vi "save file data.vi"(8 "error in":errorcluster, 10 "format":T1, 11 "Path":path) -> (0 "error out":errorcluster)   [LabVIEW 2013, in "NISE_CEF_TreeSerializer.lvlib"]
uses:
  NISE_CEF_TreeSerializer.lvlib
  base file format.ctl
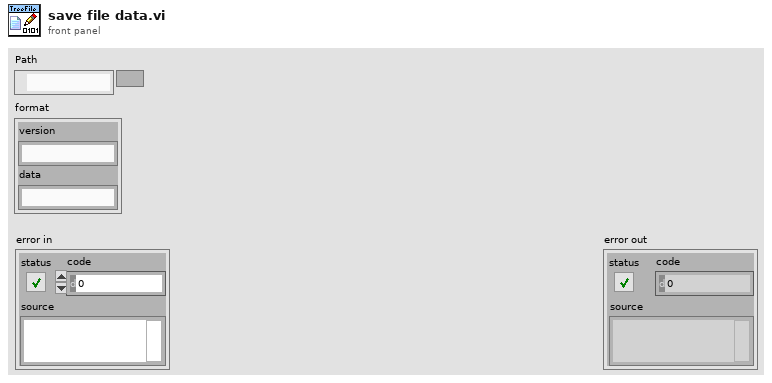
[diagram p1: front panel]
types:
  T1 = typedef "NISE_CEF_TreeSerializer.lvlib/base file format.ctl" = cluster{"version":string, "data":string}
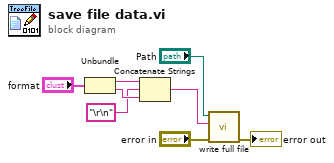
[diagram p0: block diagram]
diagram:
  n1 = Unbundle("format") -> ("version"=w6:string, "data"=w7:string)
  n2 = Concatenate Strings(w6, "\r\n" ("String"), w7) -> (w4:string)
  n3 = call "write full file.vi"("error in"="error in", "data"=w4, "file path"="Path") -> ("error out"=→"error out":errorcluster)  [unwired: 8 in]
